vi "Trigger Send File.vi"() -> ()   [LabVIEW 2016]
uses:
  <vilib>/Message/Open (Sync).vi
  <vilib>/Message/Publish (Sync).vi
  <vilib>/Message/Close (Sync).vi
  <vilib>/Message/Message.lvlib
panel:
  out "error out":errorcluster
  in  "topic":string="send_file"
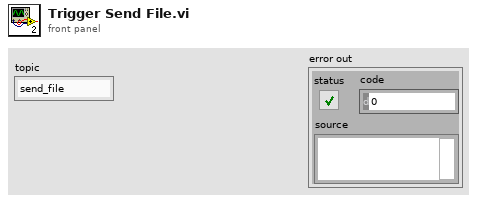
[diagram p1: front panel]
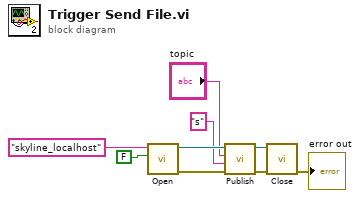
[diagram p0: block diagram]
diagram:
  n1 = call-poly <vilib>:"Open.vi"("Enable Fallbacks (T)"=FALSE, "Skyline Configuration Id"="skyline_localhost") -> ("error out"=w8:errorcluster, "message sync reference"=w9:refnum<k21>)  [unwired: 8 in]
  n2 = call-poly <vilib>:"Publish.vi"("error in (no error)"=w8, "message"="s", "topic"="topic", "message sync reference in"=w9) -> ("error out"=w6:errorcluster, "message sync reference out"=w7:refnum<k21>)  [unwired: 6 in]
  n3 = call-poly <vilib>:"Close.vi"("error in"=w6, "message sync reference"=w7) -> ("error out"=→"error out":errorcluster)  [unwired: 9 in]
